vi "Format Gas Params Refactored.vi"() -> ()   [LabVIEW 2014]
panel:
  in  "error in":errorcluster
  out "error out":errorcluster
  out "Result":string
  in  "Gas Parameter Names":string[](array[string])=["Temperature", "Pressure", "Humidity", "Volume", "Density"]
  in  "Gas Parameter Values":dbl[](array[numeric])=[1.0, 2.0, 3.0, 4.0, 5.0]
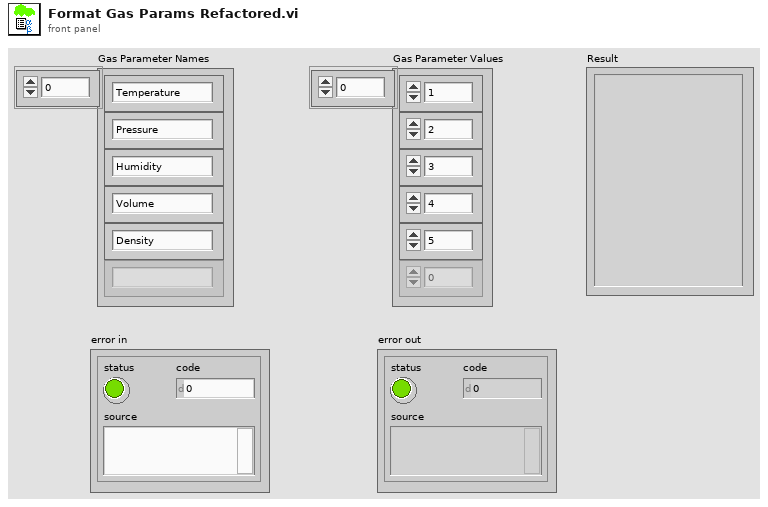
[diagram p1: front panel]
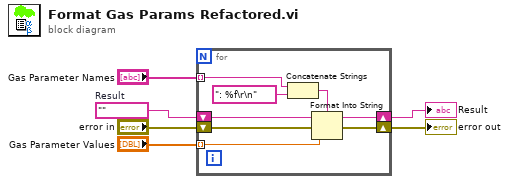
[diagram p0: block diagram]
diagram:
  w3 = ""  # Result
  n1 = for {
    tunnel: "Gas Parameter Values" -> [w7] mode=indexing
    shift-right: [w9] -> w4
    shift-left: w3 -> [w10]
    tunnel: "Gas Parameter Names" -> [w14] mode=indexing
    shift-right: [w11] -> w2
    shift-left: "error in" -> [w8]
    n2 = Concatenate Strings(w14, ": %f\r\n" ("string")) -> (w12:string)
    n3 = Format Into String(format string=w12, initial string=w10, error in=w8, w7) -> (resulting string=w9:string, error out=w11:errorcluster)
  }
  "Result" <- w4
  "error out" <- w2
